vi "GetChartContent.vi"(0 "reference in":refnum<class "LcWebView.lvclass">, 1 "Chart Id":string, 5 "error in (no error)":errorcluster) -> (14 "reference out":refnum<class "LcWebView.lvclass">, 15 "Chart Content":T1, 19 "error out":errorcluster)   [LabVIEW 2018, in "LcWebView.lvclass"]
uses:
  LcWebView.lvclass
  ctrls/ChartContent.ctl
  ctrls/ChartSetup.ctl
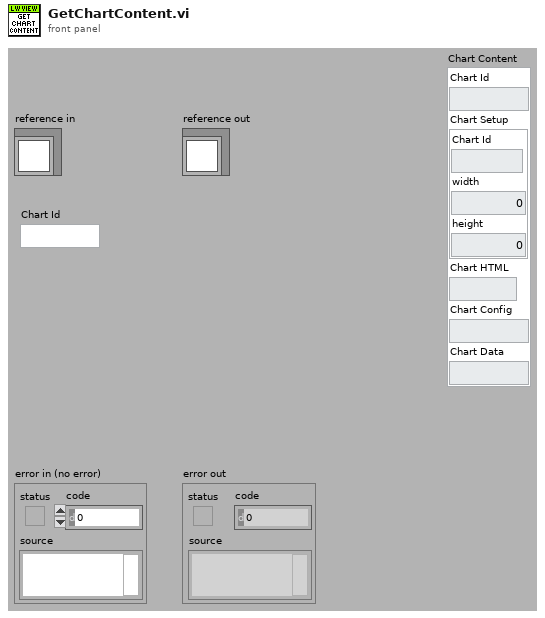
[diagram p1: front panel]
types:
  T1 = typedef "LcWebView.lvclass/ChartContent.ctl" = cluster{"Chart Id":string, "Chart Setup":T2, "Chart HTML":string, "Chart Config":string, "Chart Data":string}
  T2 = typedef "LcWebView.lvclass/ChartSetup.ctl" = cluster{"Chart Id":string, "width":u32, "height":u32}
  T3 = typedef "LcWebView.lvclass/ObjectAttributes.ctl" = cluster{"WebView Container":refnum<k24>, "CoreWebViewRef":refnum<k24>, "Status":i32, "Status Message":string, "User Data Folder":path, "BrowserProcessId":u32, "PlotType":T4, "Chart Collection":T5}
  T4 = typedef "LcWebView.lvclass/PlotType.ctl" = enum16{"bar", "line", "pie"}
  T5 = typedef "LcWebView.lvclass/ChartCollection.ctl" = T1[]
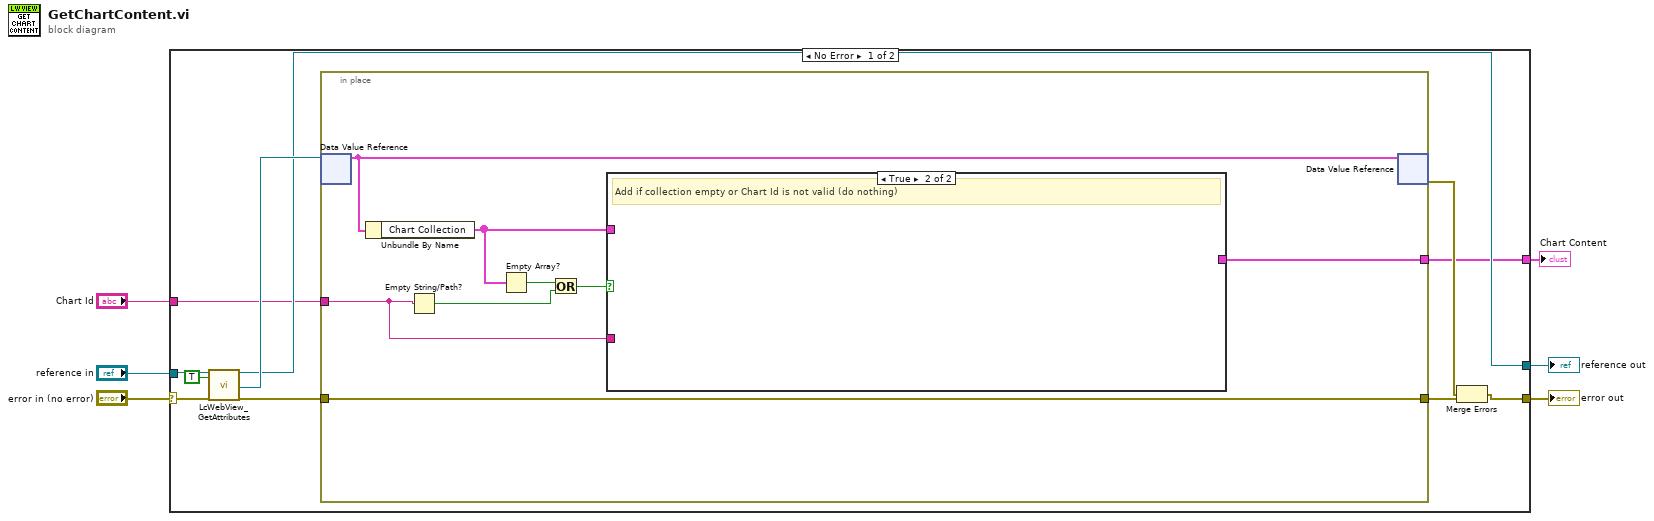
[diagram p0: block diagram]
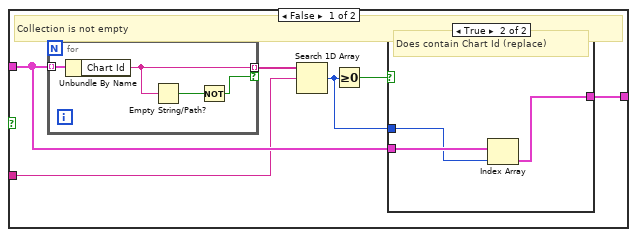
[diagram p2: hidden frame]
diagram:
  n1 = case shown="No Error" "error in (no error)" {
    selector: "error in (no error)" -> [w17 w40]
    tunnel: [w9 w40] -> w5
    tunnel: [w12 w39] -> w3
    tunnel: "reference in" -> [w16 w39]
    tunnel: "Chart Id" -> [w8 _]
    tunnel: [w7 _] -> w1
    frame No Error {
      n2 = call "LcWebView_GetAttributes.vi"("reference in"=w16, "OnlyGetDvrReference(False)"=TRUE, "error in (no error)"=w17) -> ("reference out"=w12:refnum<class "LcWebView.lvclass">, "DataRef"=w15:refnum<data-value>, "error out"=w13:errorcluster)  [unwired: 13 in, 1 out]
      n3 = in-place {
        in-place-border: w13 -> [w24]
        in-place-border: [w24] -> w11
        in-place-border: w8 -> [w20]
        in-place-border: [w19] -> w7
        n4 = in-place-dvr #1(w15) -> (w18:T3)  [unwired: 1 out]
        n5 = Unbundle By Name(w18) -> ("Chart Collection"=w25:T5)
        n6 = Empty String/Path?(string/path=w20) -> (empty?=w23:bool)
        n7 = Empty Array?(array=w25) -> (empty?=w22:bool)
        n8 = Or(x=w22, y=w23) -> (x .or. y?=w21:bool)
        n9 = case shown="True" w21 {
          tunnel: w25 -> [w29 _]
          tunnel: w20 -> [w27 _]
          tunnel: [w26 _] -> w19
          frame False {
            # "Collection is not empty"
            n10 = for {
              tunnel: w29 -> [w38] mode=indexing
              tunnel: [w37] -> w31 mode=indexing if=w35
              n11 = Unbundle By Name(w38) -> ("Chart Id"=w37:string)
              n12 = Empty String/Path?(string/path=w37) -> (empty?=w36:bool)
              n13 = Not(x=w36) -> (.not. x?=w35:bool)
            }
            n14 = Search 1D Array(1D array=w31, element=w27) -> (index of element=w28:i32)  [unwired: 1 in]
            n15 = Greater Or Equal To 0?(x=w28) -> (x >= 0?=w30:bool)
            n16 = case shown="True" w30 {
              tunnel: w29 -> [_ w34]
              tunnel: w28 -> [_ w33]
              tunnel: [_ w32] -> w26
              frame False {
                # "Does not contain (do nothing)"
              }
              frame True {
                # "Does contain Chart Id (replace)"
                n17 = Index Array(array=w34, index=w33) -> (element=w32:T1)
              }
            }
          }
          frame True {
            # "Add if collection empty or Chart Id is not valid (do nothing)"
          }
        }
        n18 = in-place-dvr #1(w18) -> (w10:errorcluster)  [unwired: 1 out]
      }
      n19 = Merge Errors(w10, w11) -> (w9:errorcluster)
    }
    frame Error {
    }
  }
  "error out" <- w5
  "reference out" <- w3
  "Chart Content" <- w1
